vi "Method.vi"(4 "Input B":refnum<class "Abs_Numeric.lvclass">, 5 "Input A":T1) -> (1 "Result":T1)   [LabVIEW 2021, in "Multiply_I32.lvclass"]
uses:
  Multiply_I32.lvclass
  Abs_Type.ctl
  Abs_Types/I32 Integer/Abs_I32 Integer.lvclass
  Abs_Types/Numeric/Abs_Numeric.lvclass
  C:/Users/Tim/Documents/LabVIEW/2021/Data Classes/Source/Functions/Support/Two Terminal/I32/AbsFunc_Two Term_I32.lvclass
  C:/Users/Tim/Documents/LabVIEW/2021/Data Classes/Source/Abs_Types/I32 Integer/Abs_I32 Integer.lvclass
  Support/Two Terminal/I32/AbsFunc_Two Term_I32.lvclass/AbsFunc_Two Term_I32.ctl
  Support/Two Terminal/I32/Properties/Write Numeric A.vi
  Support/Two Terminal/I32/Properties/Write Numeric B.vi
  Multiply_I32.lvclass/Multiply_I32.ctl
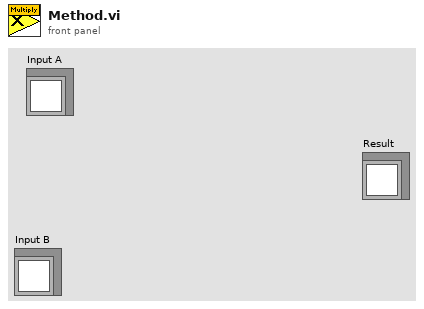
[diagram p1: front panel]
types:
  T1 = typedef "Multiply_I32.lvclass/Abs_Type.ctl" = refnum<class "Abs_I32 Integer.lvclass">
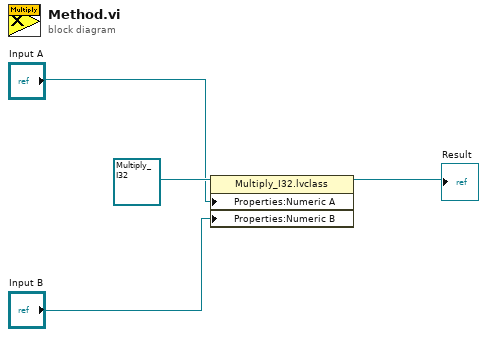
[diagram p0: block diagram]
diagram:
  n1 = property class="Multiply_I32.lvclass"(reference=refnum<class "Multiply_I32.lvclass"> refnum ("Functions.lvlib:Numeric.lvlib:Multiply.lvclass"), "Properties:Numeric A"="Input A", "Properties:Numeric B"="Input B") -> (reference out=→"Result":refnum<class "Multiply_I32.lvclass">)  [unwired: 1 in, 1 out]
